vi "azimuth_angle.vi"(1 "Time (h of day)":dbl, 2 "Day of Year (day)":dbl, 3 "Latitude (rad)":dbl) -> (0 "Solar Azimuth (rad)":dbl)   [LabVIEW 2012]
panel:
  out "Solar Azimuth (¼)":dbl
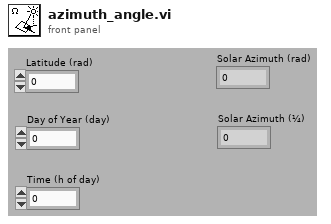
[diagram p1: front panel]
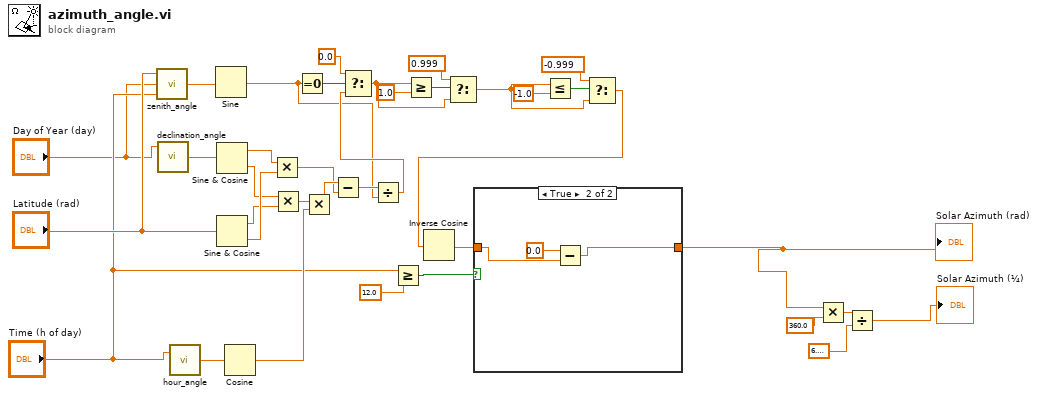
[diagram p0: block diagram]
diagram:
  n1 = call "zenith_angle.vi"("Time (hour of day)"="Time (h of day)", "Day of Year (day)"="Day of Year (day)", "Latitude (rad, +:N, -:S)"="Latitude (rad)") -> ("Zenith angle (rad)"=w27:dbl)
  n2 = call "declination_angle.vi"("Day of Year (day)"="Day of Year (day)") -> ("Declination (rad)"=w1:dbl)  [unwired: 2 in]
  n3 = call "hour_angle.vi"("Time (hour of day since midnight)"="Time (h of day)") -> ("Hour angle h (rad)"=w3:dbl)  [unwired: 1 in]
  n4 = Sine(x=w27) -> (sin(x)=w14:dbl)
  n5 = Sine & Cosine(0:w1) -> (1:w31:dbl, 2:w28:dbl)
  n6 = Sine & Cosine(0:"Latitude (rad)") -> (1:w29:dbl, 2:w30:dbl)
  n7 = Cosine(x=w3) -> (cos(x)=w35:dbl)
  n8 = Multiply(x=w31, y=w30) -> (x*y=w20:dbl)
  n9 = Multiply(x=w28, y=w29) -> (x*y=w36:dbl)
  n10 = Equal To 0?(x=w14) -> (x = 0?=w17:bool)
  n11 = Multiply(x=w36, y=w35) -> (x*y=w21:dbl)
  n12 = Subtract(x=w21, y=w20) -> (x-y=w34:dbl)
  n13 = Divide(x=w34, y=w14) -> (x/y=w15:dbl)
  n14 = Select(t=0.0, s=w17, f=w15) -> (s? t:f=w11:dbl)
  n15 = Greater Or Equal?(x="Time (h of day)", y=12.0) -> (x >= y?=w33:bool)
  n16 = Greater Or Equal?(x=w11, y=1.0) -> (x >= y?=w12:bool)
  n17 = Select(t=0.999, s=w12, f=w11) -> (s? t:f=w6:dbl)
  n18 = Less Or Equal?(x=w6, y=-1.0) -> (x <= y?=w8:bool)
  n19 = Select(t=-0.999, s=w8, f=w6) -> (s? t:f=w5:dbl)
  n20 = Inverse Cosine(1:w5) -> (0:w18:dbl)
  n21 = case shown="True" w33 {
    tunnel: w18 -> [w37 w40]
    tunnel: [w37 w38] -> w19
    frame False {
    }
    frame True {
      n22 = Subtract(x=0.0, y=w40) -> (x-y=w38:dbl)
    }
  }
  "Solar Azimuth (rad)" <- w19
  n23 = Multiply(x=w19, y=360.0) -> (x*y=w24:dbl)
  n24 = Divide(x=w24, y=6.283185307179586) -> (x/y=→"Solar Azimuth (¼)":dbl)
